vi "get all classes from packed library.vi"(8 "error in":errorcluster, 11 "packed library path":path) -> (0 "error out":errorcluster, 2 "all class names[]":string[](array[string]), 3 "all classes path":path[](array[path]))   [LabVIEW 2020, in "Reusable Library.lvlib"]
uses:
  <userlib>/_Reusable Library/Reusable Library.lvlib
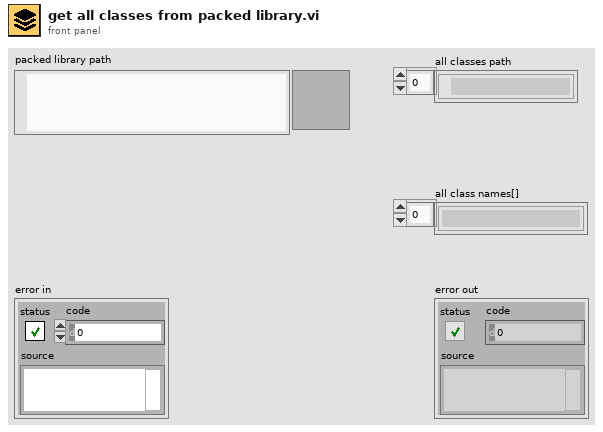
[diagram p1: front panel]
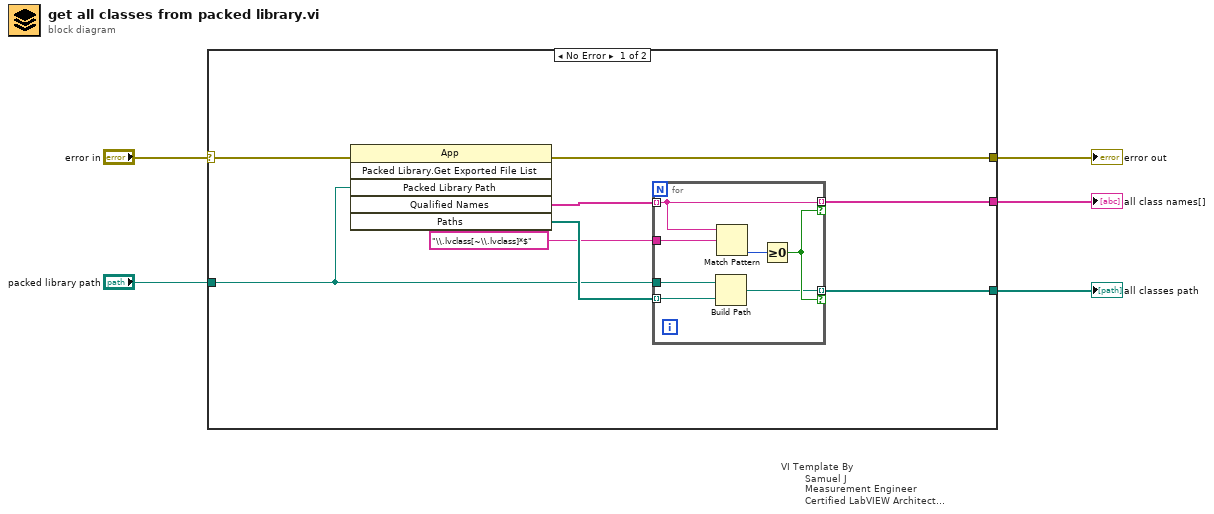
[diagram p0: block diagram]
diagram:
  n1 = case "VI Template By\n        Samuel J\n        Measurement Engineer\n        Certified LabVIEW Architect\n        Vestas Technology R&D Chennai" shown="No Error" "error in" {
    selector: "error in" -> [w10 w21]
    tunnel: "packed library path" -> [w9 _]
    tunnel: [w8 w21] -> w3
    tunnel: [w7 _] -> w2
    tunnel: [w6 _] -> w1
    frame No Error {
      n2 = invoke class="App" method="Packed Library.Get Exported File List"(error in=w10, "Packed Library Path"=w9) -> (error out=w8:errorcluster, "Qualified Names"=w12:string[], "Paths"=w13:path[])  [unwired: 4 in, 3 out]
      n3 = for {
        tunnel: "\\.lvclass[~\\.lvclass]*$" ("regular expression") -> [w20]
        tunnel: w12 -> [w18] mode=indexing
        tunnel: [w15] -> w6 mode=indexing if=w17
        tunnel: w13 -> [w14] mode=indexing
        tunnel: [w18] -> w7 mode=indexing if=w17
        tunnel: w9 -> [w16]
        n4 = Build Path(base path=w16, name or relative path=w14) -> (appended path=w15:path)
        n5 = Match Pattern(string=w18, regular expression=w20) -> (offset past match=w19:i32)  [unwired: 4 out]
        n6 = Greater Or Equal To 0?(x=w19) -> (x >= 0?=w17:bool)
      }
    }
    frame Error {
    }
  }
  "all classes path" <- w1
  "all class names[]" <- w2
  "error out" <- w3
